vi "Config File Path.vi"(1 "AppName":string) -> (0 "Default config file name":path)   [LabVIEW 2020]
uses:
  <vilib>/Utility/sysdir.llb/System Directory Type.ctl
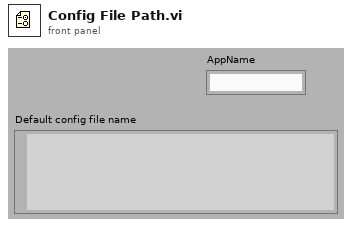
[diagram p1: front panel]
types:
  T1 = typedef "System Directory Type.ctl" = i32
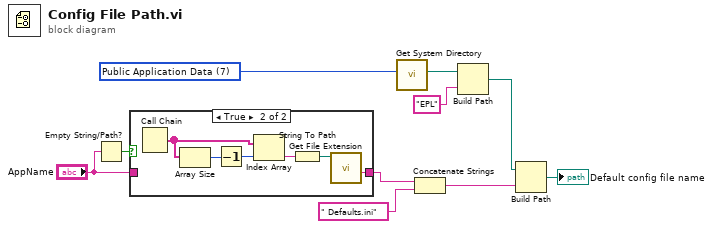
[diagram p0: block diagram]
diagram:
  w7 = T1 7 items=["User Home", "User Desktop", "User Documents", "User Application Data", "User Preferences", "User Temporary", "Public Documents", "Public Application Data", "Public Preferences", "System Core Libraries", "System Installed Libraries", "Application Files", "Boot Volume Root"] ("system directory type")
  n1 = Empty String/Path?(string/path="AppName") -> (empty?=w2:bool)
  n2 = case shown="True" w2 {
    tunnel: [w11 w12] -> w3
    tunnel: "AppName" -> [w11 _]
    frame False {
    }
    frame True {
      n3 = Call Chain() -> (call chain=w17:string[])
      n4 = Array Size(array=w17) -> (size(s)=w16:i32)
      n5 = Decrement(x=w16) -> (x-1=w15:i32)
      n6 = Index Array(array=w17, index=w15) -> (element=w13:string)
      n7 = String To Path(string=w13) -> (path=w14:path)
      n8 = call <vilib>:"Get File Extension.vi"("file"=w14) -> ("filename without extension"=w12:string)  [unwired: 6 in, 4 out]
    }
  }
  n9 = call <vilib>:"Get System Directory.vi"("system directory type"=w7) -> ("system directory"=w6:path)  [unwired: 10 in]
  n10 = Concatenate Strings(w3, " Defaults.ini" ("string")) -> (w8:string)
  n11 = Build Path(base path=w6, name or relative path="EPL") -> (appended path=w5:path)
  n12 = Build Path(base path=w5, name or relative path=w8) -> (appended path=→"Default config file name":path)
